vi "Radio Buttons - Entire Dataset for desired quantity + save.vi"() -> ()   [LabVIEW 2020]
panel:
  in  "File Name Txt Version 2":string
  in  "Folder to Save Data - Txt Version 2":path
  in  "File Name A-Scan ASCII":string
  in  "Folder to Save Data - A-Scan ASCII":path
  in  "Format String A-Scan ASCII":string
  in  "File Name A-Scan CSV":string
  in  "Folder to Save Data - A-Scan CSV":path
  in  "Format String A-Scan CSV":string
  in  "File Name A-Scan":string
  in  "Folder to Save Data - A-Scan":path
  in  "Format String A-Scan":string
  in  "File Name - DQ":string
  in  "Folder to Save Data -DQ":path
  in  "Format String -DQ":string
  out "XY Graph":cluster{dbl[], dbl[]}(graph)
  out "output array":dbl[][](array[numeric])
  out "Intensity Graph":dbl[][](graph)
  in  "Radio Buttons":T1(radio)=enum."Peak Positive"
  in  "Rows":dbl
  in  "Columns":dbl
  in  "Input Data Path":path=path "C:/Users/gaeta/Desktop/Unif Leerstof/Individual Project/Osc. Data/wetransfer-86c2d3/2DZXaxisscan 0.28MHz 30x30mm 20mvpp 1020L centre 390mm from td plane.mat"
  # "%f - float\n%d - digit"
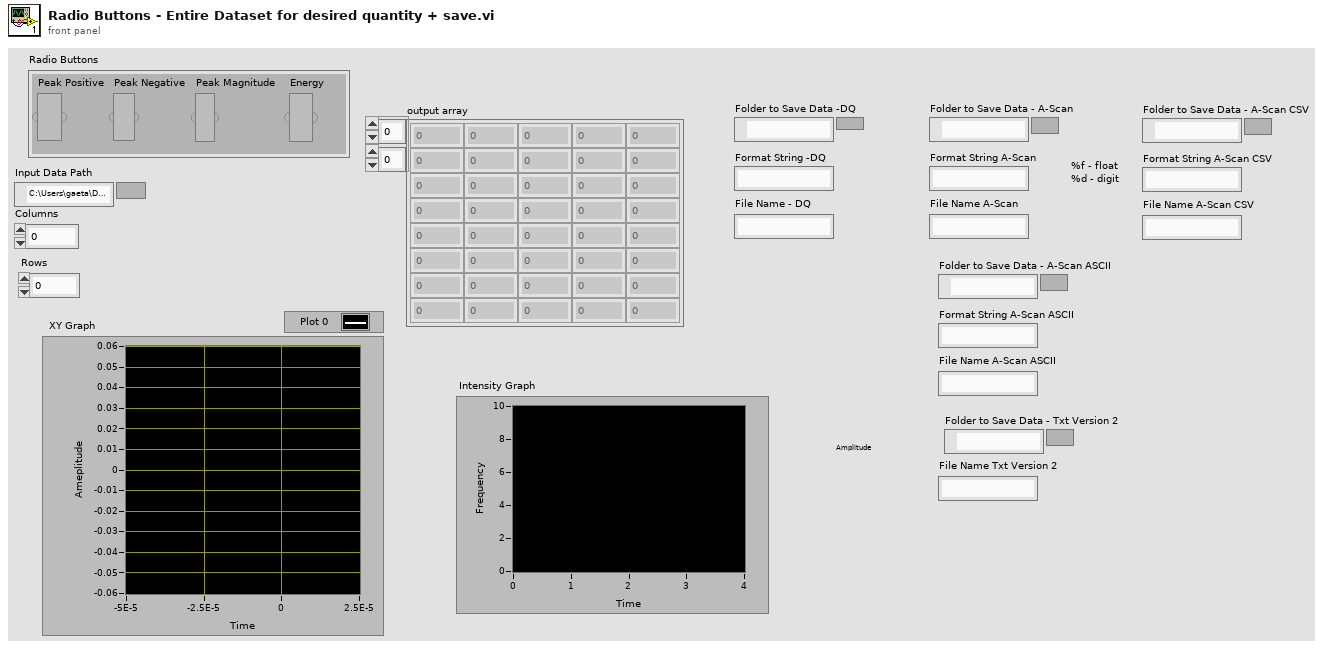
[diagram p1: front panel]
types:
  T1 = enum32{"No Selection", "Peak Positive", "Peak Negative", "Peak Magnitude", "Energy"}
  T2 = enum16{"open", "replace", "create", "open or create", "replace or create", "replace or create with confirmation"}
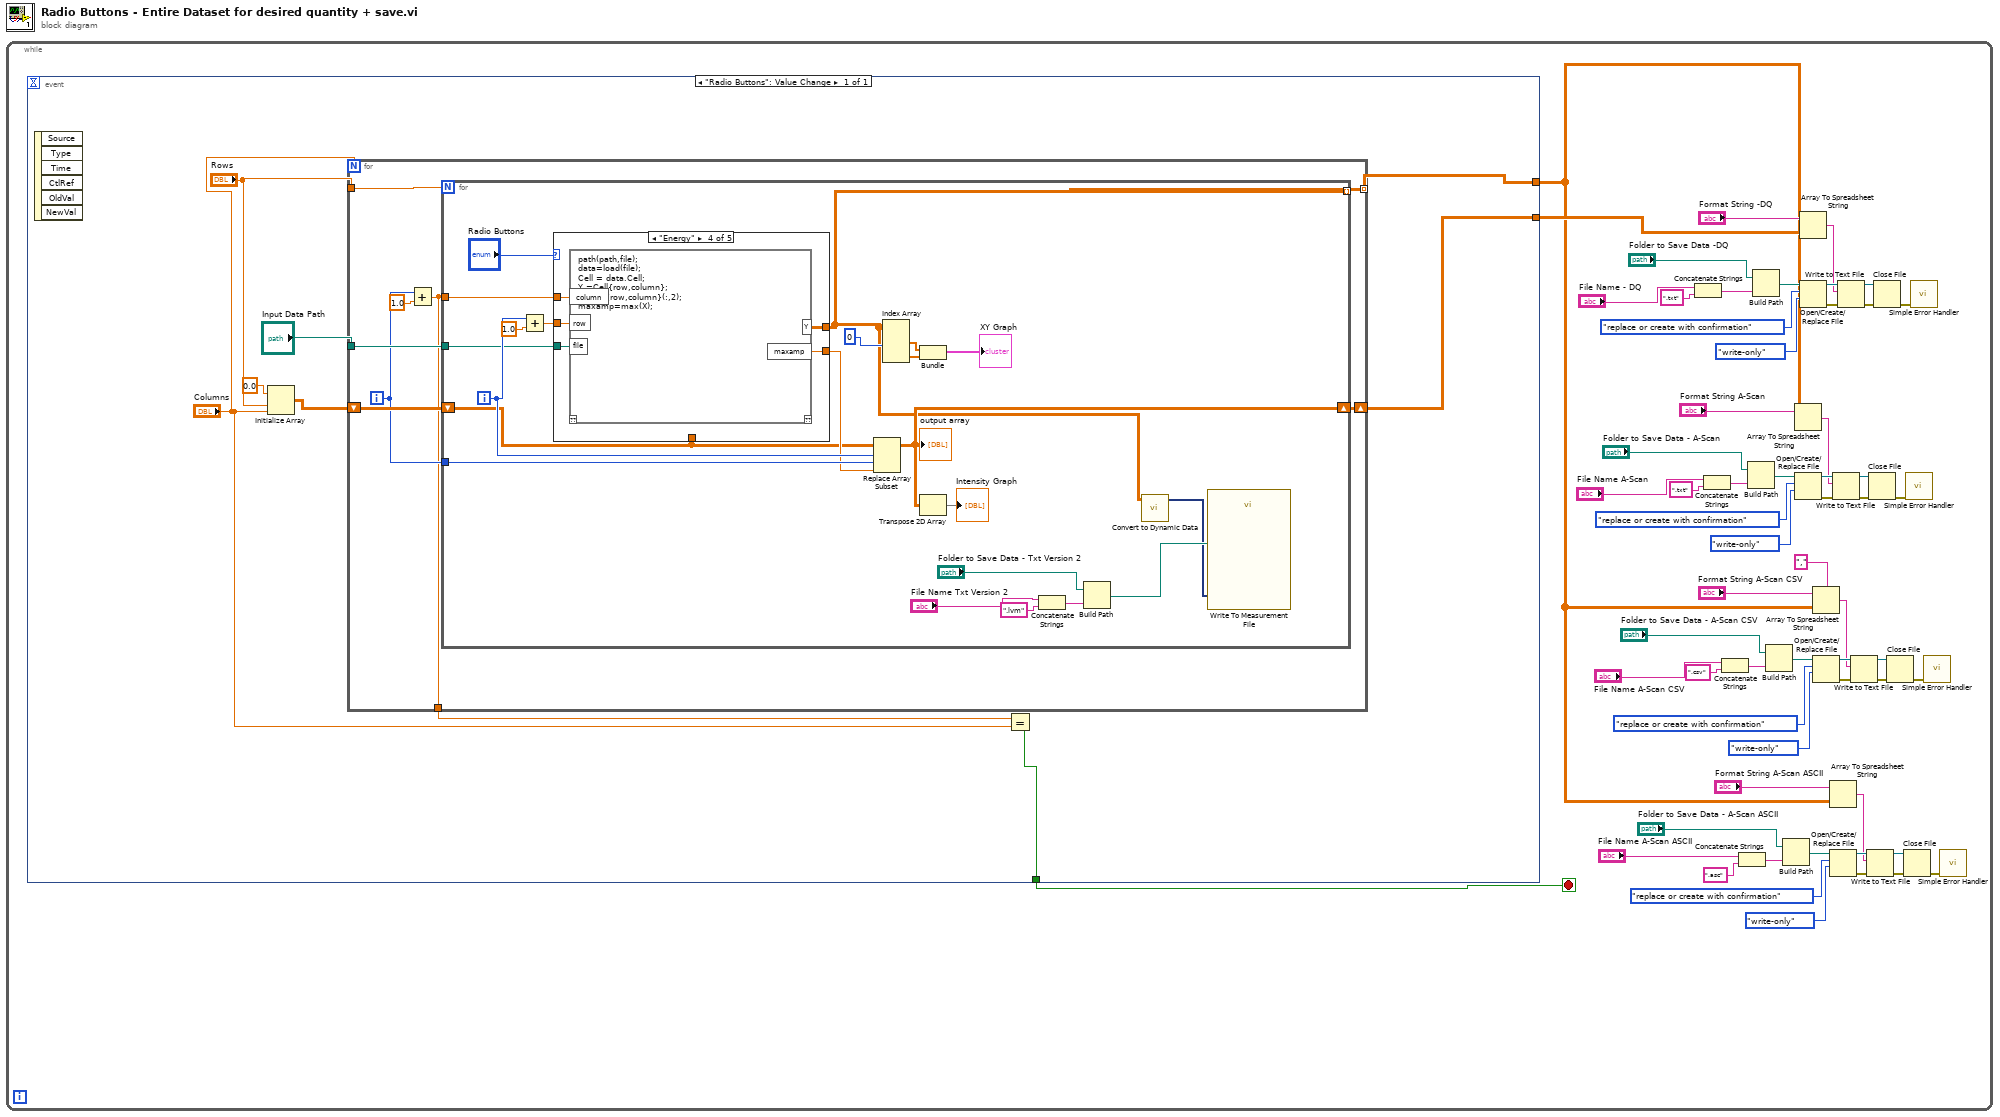
[diagram p0: block diagram]
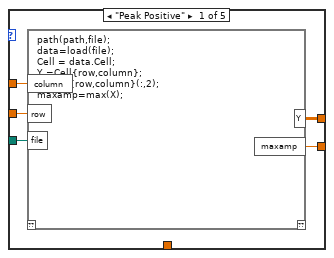
[diagram p2: hidden frame]
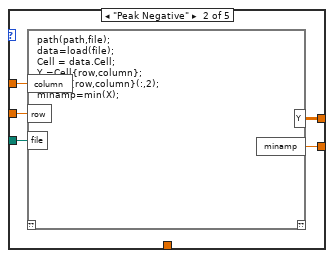
[diagram p3: hidden frame]
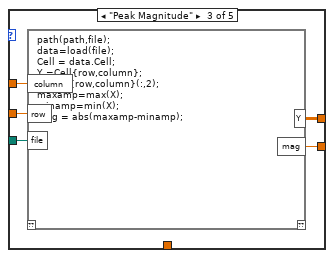
[diagram p4: hidden frame]
diagram:
  n1 = while {
    stop <- w31 stop-if-true
    n2 = event shown="[0] \"Radio Buttons\": Value Change" {
      selector: _ -> [_]
      dyn-events: _ -> [_]
      timeout: _ -> [_]
      tunnel: [w63] -> w31
      tunnel: [w62] -> w52
      tunnel: [w61] -> w1
      event "Radio Buttons": Value Change {
        n3 = event-data() -> ()  [unwired: 1 in, 6 out]
        n4 = Initialize Array(0.0 ("element"), "Rows", "Columns") -> (w66:dbl[][])
        n5 = for {
          N: "Columns" -> [_]
          tunnel: "Input Data Path" -> [w77]
          tunnel: "Rows" -> [w75]
          shift-right: [w73] -> w62
          shift-left: w66 -> [w74]
          tunnel: [w71] -> w64
          tunnel: [w70] -> w61 mode=indexing
          i -> [w72]
          n6 = Add(x=w72, y=1.0) -> (x+y=w71:dbl)
          n7 = for {
            N: w75 -> [_]
            tunnel: w77 -> [w90]
            tunnel: w71 -> [w92]
            shift-right: [w85] -> w73
            shift-left: w74 -> [w88]
            tunnel: w72 -> [w93]
            tunnel: [w78] -> w70 mode=indexing
            i -> [w95]
            n8 = Add(x=w95, y=1.0) -> (x+y=w91:dbl)
            n9 = case shown="\"Energy\"" "Radio Buttons" {
              tunnel: w92 -> [w100 w105 w110 w115 _]
              tunnel: w91 -> [w104 w109 w112 w117 _]
              tunnel: w90 -> [w103 w108 w111 w116 _]
              tunnel: [w101 w107 w113 w118 _] -> w89
              tunnel: [w102 w106 w114 w119 _] -> w78
              tunnel: w88 -> [_ _ _ _ _]
              frame "Peak Positive" {
                n10 = script code="path(path,file);\ndata=load(file);\nCell = data.Cell;\nY =Cell{row,column};\nX=Cell{row,column}(:,2);\nmaxamp=max(X);"("row"=w104, "file"=w103, "column"=w100) -> ("Y"=w102:dbl[][], "maxamp"=w101:dbl)  [unwired: 1 in, 1 out]
              }
              frame "Peak Negative" {
                n11 = script code="path(path,file);\ndata=load(file);\nCell = data.Cell;\nY =Cell{row,column};\nX=Cell{row,column}(:,2);\nminamp=min(X);"("row"=w109, "file"=w108, "column"=w105) -> ("Y"=w106:dbl[][], "minamp"=w107:dbl)  [unwired: 1 in, 1 out]
              }
              frame "Peak Magnitude" {
                n12 = script code="path(path,file);\ndata=load(file);\nCell = data.Cell;\nY =Cell{row,column};\nX=Cell{row,column}(:,2);\nmaxamp=max(X);\nminamp=min(X);\nmag = abs(maxamp-minamp);"("row"=w112, "file"=w111, "column"=w110) -> ("Y"=w114:dbl[][], "mag"=w113:dbl)  [unwired: 1 in, 1 out]
              }
              frame "Energy" {
                n13 = script code="path(path,file);\ndata=load(file);\nCell = data.Cell;\nY =Cell{row,column};\nX=Cell{row,column}(:,2);\nmaxamp=max(X);"("row"=w117, "file"=w116, "column"=w115) -> ("Y"=w119:dbl[][], "maxamp"=w118:dbl)  [unwired: 1 in, 1 out]
              }
              frame "No Selection" {
              }
            }
            n14 = Replace Array Subset(array=w88, new element=w89, index (row)=w95, index (col)=w93) -> (w85:dbl[][])
            "output array" <- w85
            n15 = Index Array(array=w78, index (col) #1=0 ("disabled index (col)")) -> (element #1=w97:dbl[], element #2=w98:dbl[])  [unwired: 3 in]
            n16 = Bundle(w97, w98) -> (→"XY Graph":cluster{dbl[], dbl[]})  [unwired: 1 in]
            n17 = Transpose 2D Array(2D array=w85) -> (transposed array=→"Intensity Graph":dbl[][])
            n18 = Concatenate Strings("File Name Txt Version 2", ".lvm" ("string")) -> (w83:string)
            n19 = Build Path(base path="Folder to Save Data - Txt Version 2", name or relative path=w83) -> (appended path=w84:path)
            n20 = call "Convert to Dynamic Data"("2D Array"=w78) -> ("Dynamic Data Type"=w79:dynamicdata)  [unwired: 3 in]
            n21 = call "Write To Measurement File"("Signals"=w79, "Filename"=w84) -> ()  [unwired: 15 in, 3 out]
          }
        }
        n22 = Equal?(x=w64, y="Columns") -> (x = y?=w63:bool)
      }
    }
    n23 = Concatenate Strings("File Name - DQ", ".txt" ("string")) -> (w50:string)
    n24 = Concatenate Strings("File Name A-Scan", ".txt" ("string")) -> (w38:string)
    n25 = Concatenate Strings("File Name A-Scan CSV", ".csv" ("string")) -> (w23:string)
    n26 = Concatenate Strings("File Name A-Scan ASCII", ".asc" ("string")) -> (w8:string)
    n27 = Build Path(base path="Folder to Save Data - A-Scan", name or relative path=w38) -> (appended path=w36:path)
    n28 = Build Path(base path="Folder to Save Data -DQ", name or relative path=w50) -> (appended path=w48:path)
    n29 = Build Path(base path="Folder to Save Data - A-Scan CSV", name or relative path=w23) -> (appended path=w21:path)
    n30 = Build Path(base path="Folder to Save Data - A-Scan ASCII", name or relative path=w8) -> (appended path=w6:path)
    n31 = Array To Spreadsheet String(array=w1, 3:"Format String A-Scan") -> (spreadsheet string=w32:string)  [unwired: 1 in]
    n32 = Open/Create/Replace File(file path (use dialog)=w36, operation (0:open)=T2."replace or create with confirmation", access (0:read/write)=enum16{"read/write", "read-only", "write-only"}."write-only") -> (refnum out=w43:refnum<file>, error out=w44:errorcluster)  [unwired: 1 in, 3 out]
    n33 = Array To Spreadsheet String(array=w52, 3:"Format String -DQ") -> (spreadsheet string=w51:string)  [unwired: 1 in]
    n34 = Open/Create/Replace File(file path (use dialog)=w48, operation (0:open)=T2."replace or create with confirmation", access (0:read/write)=enum16{"read/write", "read-only", "write-only"}."write-only") -> (refnum out=w57:refnum<file>, error out=w58:errorcluster)  [unwired: 1 in, 3 out]
    n35 = Array To Spreadsheet String(delimiter (Tab)=",", array=w1, 3:"Format String A-Scan CSV") -> (spreadsheet string=w17:string)
    n36 = Open/Create/Replace File(file path (use dialog)=w21, operation (0:open)=T2."replace or create with confirmation", access (0:read/write)=enum16{"read/write", "read-only", "write-only"}."write-only") -> (refnum out=w28:refnum<file>, error out=w29:errorcluster)  [unwired: 1 in, 3 out]
    n37 = Array To Spreadsheet String(array=w1, 3:"Format String A-Scan ASCII") -> (spreadsheet string=w3:string)  [unwired: 1 in]
    n38 = Open/Create/Replace File(file path (use dialog)=w6, operation (0:open)=T2."replace or create with confirmation", access (0:read/write)=enum16{"read/write", "read-only", "write-only"}."write-only") -> (refnum out=w13:refnum<file>, error out=w14:errorcluster)  [unwired: 1 in, 3 out]
    n39 = Write to Text File(file (use dialog)=w43, text=w32, error in=w44) -> (refnum out=w40:refnum<file>, error out=w41:errorcluster)  [unwired: 1 in, 1 out]
    n40 = Write to Text File(file (use dialog)=w57, text=w51, error in=w58) -> (refnum out=w54:refnum<file>, error out=w55:errorcluster)  [unwired: 1 in, 1 out]
    n41 = Write to Text File(file (use dialog)=w28, text=w17, error in=w29) -> (refnum out=w25:refnum<file>, error out=w26:errorcluster)  [unwired: 1 in, 1 out]
    n42 = Write to Text File(file (use dialog)=w13, text=w3, error in=w14) -> (refnum out=w10:refnum<file>, error out=w11:errorcluster)  [unwired: 1 in, 1 out]
    n43 = Close File(refnum=w40, error in=w41) -> (error out=w45:errorcluster)  [unwired: 1 out]
    n44 = Close File(refnum=w54, error in=w55) -> (error out=w59:errorcluster)  [unwired: 1 out]
    n45 = Close File(refnum=w25, error in=w26) -> (error out=w30:errorcluster)  [unwired: 1 out]
    n46 = Close File(refnum=w10, error in=w11) -> (error out=w15:errorcluster)  [unwired: 1 out]
    n47 = call <vilib>:"Simple Error Handler.vi"("error in (no error)"=w45) -> ()  [unwired: 1 in, 8 out]
    n48 = call <vilib>:"Simple Error Handler.vi"("error in (no error)"=w59) -> ()  [unwired: 1 in, 8 out]
    n49 = call <vilib>:"Simple Error Handler.vi"("error in (no error)"=w30) -> ()  [unwired: 1 in, 8 out]
    n50 = call <vilib>:"Simple Error Handler.vi"("error in (no error)"=w15) -> ()  [unwired: 1 in, 8 out]
  }
